vi "60pt Mov Avg.vi"(10 "Value in":dbl) -> (2 "Value out":dbl)   [LabVIEW 2014]
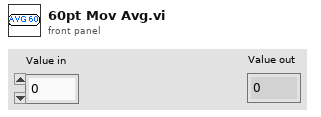
[diagram p1: front panel]
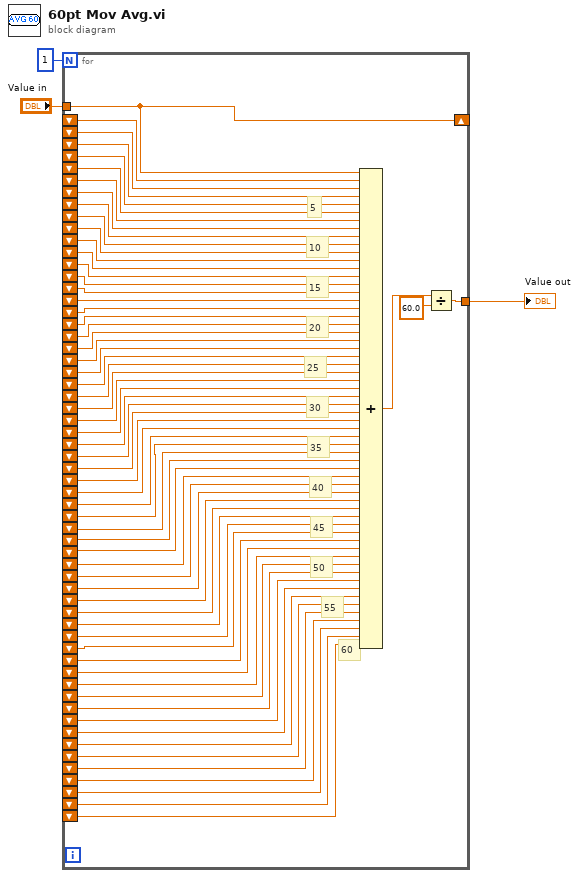
[diagram p0: block diagram]
diagram:
  n1 = for {
    N: 1 -> [_]
    tunnel: "Value in" -> [w66]
    shift-right: [w66] -> _
    shift-left: _ -> [w65]
    shift-left: _ -> [w64]
    shift-left: _ -> [w63]
    shift-left: _ -> [w62]
    tunnel: [w59] -> w1
    shift-left: _ -> [w58]
    shift-left: _ -> [w57]
    shift-left: _ -> [w56]
    shift-left: _ -> [w55]
    shift-left: _ -> [w54]
    shift-left: _ -> [w53]
    shift-left: _ -> [w52]
    shift-left: _ -> [w51]
    shift-left: _ -> [w50]
    shift-left: _ -> [w49]
    shift-left: _ -> [w48]
    shift-left: _ -> [w47]
    shift-left: _ -> [w46]
    shift-left: _ -> [w45]
    shift-left: _ -> [w44]
    shift-left: _ -> [w43]
    shift-left: _ -> [w42]
    shift-left: _ -> [w41]
    shift-left: _ -> [w40]
    shift-left: _ -> [w39]
    shift-left: _ -> [w38]
    shift-left: _ -> [w37]
    shift-left: _ -> [w36]
    shift-left: _ -> [w35]
    shift-left: _ -> [w34]
    shift-left: _ -> [w33]
    shift-left: _ -> [w32]
    shift-left: _ -> [w31]
    shift-left: _ -> [w30]
    shift-left: _ -> [w29]
    shift-left: _ -> [w28]
    shift-left: _ -> [w27]
    shift-left: _ -> [w26]
    shift-left: _ -> [w25]
    shift-left: _ -> [w23]
    shift-left: _ -> [w24]
    shift-left: _ -> [w22]
    shift-left: _ -> [w21]
    shift-left: _ -> [w20]
    shift-left: _ -> [w19]
    shift-left: _ -> [w18]
    shift-left: _ -> [w17]
    shift-left: _ -> [w16]
    shift-left: _ -> [w15]
    shift-left: _ -> [w14]
    shift-left: _ -> [w13]
    shift-left: _ -> [w12]
    shift-left: _ -> [w11]
    shift-left: _ -> [w10]
    shift-left: _ -> [w9]
    shift-left: _ -> [w8]
    shift-left: _ -> [w7]
    shift-left: _ -> [w6]
    shift-left: _ -> [w5]
    shift-left: _ -> [w4]
    # "55"
    # "45"
    # "35"
    # "30"
    # "25"
    # "20"
    # "15"
    # "10"
    # "5"
    # "60"
    # "50"
    # "40"
    n2 = Compound Arithmetic op=ADD(w66, w65, w64, w63, w62, w58, w57, w56, w55, w54, w53, w52, w51, w50, w49, w48, w47, w46, w45, w44, w43, w42, w41, w40, w39, w38, w37, w36, w35, w34, w33, w32, w31, w30, w29, w28, w27, w26, w25, w23, w24, w22, w21, w20, w19, w18, w17, w16, w15, w14, w13, w12, w11, w10, w9, w8, w7, w6, w5, w4) -> (w61:dbl)
    n3 = Divide(x=w61, y=60.0) -> (x/y=w59:dbl)
  }
  "Value out" <- w1
